vi "XIPIN_Adder_Subtracter_11_0.vi"   [LabVIEW 2017]
doc: "The Xilinx LogiCORE Adder Subtracter can create adders, subtracters, and adders/subtracters that operate on signed or unsigned data. In fabric, the module supports inputs ranging from 1 to 256 bits wide, and outputs ranging from 1 to 258 bits wide. I/O widths are family dependent for dsp48 implementations.\n------------------------------------\n<b>Need License</b> : No"
uses:
  <vilib>/rvi/XilinxIP/XIPIN_XNode/niFpgaXIPIN.xnode
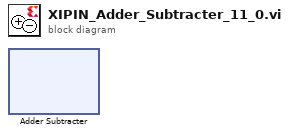
[diagram p0: block diagram]
diagram:
  n1 = xnode ("Adder Subtracter")() -> ()
